vi "Protocol.Create Protocol Settings.vi"(8 "error in (no error)":errorcluster, 10 "Name in":string, 11 "Parameters in":T4={"Name"="", "XNET.Settings"={"Database"="", "Cluster"="", "Port"="", "Baud rate [Bd]"=0, "Termination"=0, "Incoming Decimation"=0, "Outgoing Decimation"=1}, "Monitor.Network"={"Address"=0, "Name"=0, "Include DA"=FALSE}, "Data"=[], "DTCs"=[], "Sim.Nodes.LUT"=variant, "Data.LUT"=variant, "PCL"=0} {"Monitor.Network"."Name" format="%.0x"; "DTCs"."Data"."DM1.Ref"."Data Reference" format="%.0x"; "DTCs"."Data"."DM1.Enable.Ref"."Data Reference" format="%.0x"; "DTCs"."Data"."DM2.Ref"."Data Reference" format="%.0x"; "DTCs"."Data"."DM2.Enable.Ref"."Data Reference" format="%.0x"; "Data"."Trigger.Refs"."Data Reference" format="%.0x"; "Data"."Disable.Refs"."Data Reference" format="%.0x"; "Data"."Timing.Refs"."Data Reference" format="%.0x"; "Data"."Network"."Name" format="%.0x"; "Data"."Incoming.Refs"."Data Reference" format="%.0x"; "Data"."Outgoing.Refs"."Data Reference" format="%.0x"; "XNET.Settings"."Termination" items=["Off", "On"]}) -> (0 "error out":errorcluster, 3 "Protocol Refs":T1)   [LabVIEW 2019, in "J1939 Addon Engine.lvlib"]
uses:
  J1939 Addon Engine.lvlib
  Types/Protocol.App Settings.ctl
  Addon Shared/Types/XNET Settings.ctl
  Addon Shared/Types/Monitor Settings.ctl
  Types/Protocol.XNET Refs.ctl
  <vilib>/NI VeriStand/Custom Device API/Block Data Reference.ctl
  <vilib>/NI VeriStand/Custom Device API/Data Reference.ctl
  Types/Main.Outgoing.Frame.Settings.ctl
  Addon Shared/Types/Outgoing Event Trigger Types.ctl
  SubModules/Frame Protection Support/Source/Shared/Types/Exported Frame Settings.ctl
  SubModules/Frame Protection Support/Source/Shared/Types/Exported Frame Type.ctl
  SubModules/Frame Protection Support/Source/Shared/Types/Exported Protection Settings.ctl
  SubModules/Frame Protection Support/Source/Shared/Types/Protection Type.ctl
  SubModules/Frame Protection Support/Source/Shared/Types/XNET Signal Configuration.ctl
  SubModules/Frame Protection Support/Source/Shared/Types/Exported Counter Settings.ctl
  SubModules/Frame Protection Support/Source/Shared/Types/Exported Event Trigger Type.ctl
  Types/Engine.DTC Settings.ctl
  Addon Shared/Types/Compiled Simulated Settings.ctl
  Types/Engine.DTC FIFOs.ctl
  Types/Protocol.Refs.ctl
  Support Libraries/J1939 Utilities/Types/CAN Outgoing Message Cluster.ctl
  Types/Protocol.RQST Lookup Table Reference.ctl
  Types/Protocol.Address Table Reference.ctl
  Support Libraries/J1939 Utilities/J1939 Utilities.lvlib
  Addon Shared/J1939 Addon Shared.lvlib
  <vilib>/NI VeriStand/Custom Device API/Custom Device API.lvlib
  SubModules/Frame Protection Support/Source/Shared/Protection and Counter Support Shared.lvlib
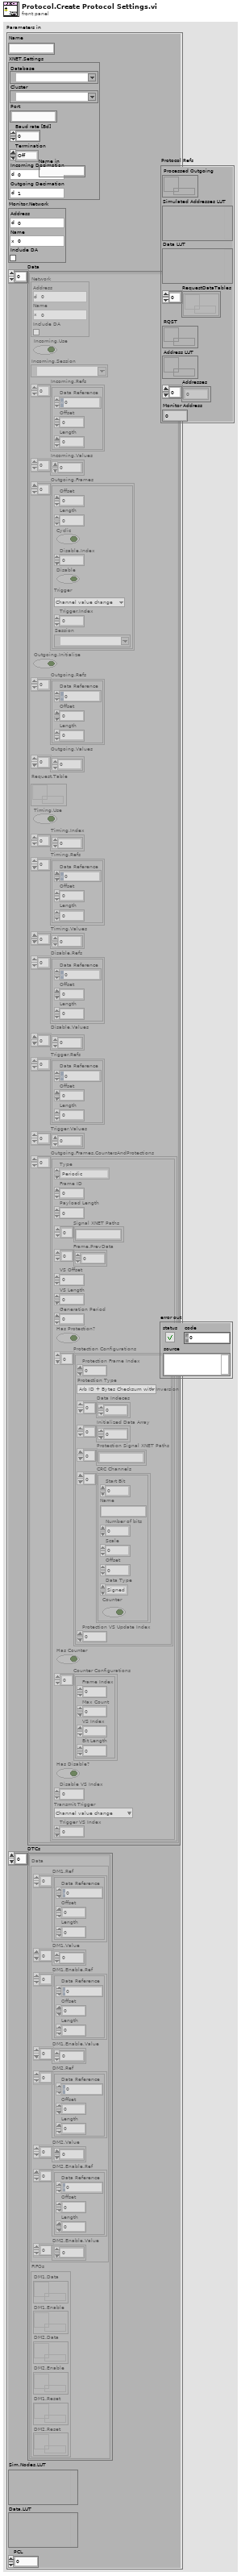
[diagram p1: front panel]
types:
  T1 = typedef "J1939 Addon Engine.lvlib/Protocol.Refs.ctl" = cluster{"Processed Outgoing":refnum<queue>, "Simulated Addresses LUT":variant, "Data LUT":variant, "RequestDataTables":refnum<k33>[], "RQST":T2, "Address LUT":T3, "Addresses":u8[], "Monitor Address":u8}
  T2 = typedef "J1939 Addon Engine.lvlib/Protocol.RQST Lookup Table Reference.ctl" = refnum<data-value>
  T3 = typedef "J1939 Addon Engine.lvlib/Protocol.Address Table Reference.ctl" = refnum<data-value>
  T4 = typedef "J1939 Addon Engine.lvlib/Protocol.App Settings.ctl" = cluster{"Name":string, "XNET.Settings":T5, "Monitor.Network":T6, "Data":T7[], "DTCs":T19[], "Sim.Nodes.LUT":variant, "Data.LUT":variant, "PCL":u32}
  T5 = typedef "J1939 Addon Shared.lvlib/XNET Settings.ctl" = cluster{"Database":refnum<k21>, "Cluster":refnum<k21>, "Port":string, "Baud rate [Bd]":u32, "Termination":u32, "Incoming Decimation":u32, "Outgoing Decimation":u32}
  T6 = typedef "J1939 Addon Shared.lvlib/Monitor Settings.ctl" = cluster{"Address":u8, "Name":u64, "Include DA":bool}
  T7 = typedef "J1939 Addon Engine.lvlib/Protocol.XNET Refs.ctl" = cluster{"Network":T6, "Incoming.Use":bool, "Incoming.Session":refnum<k21>, "Incoming.Refs":T8[], "Incoming.Values":dbl[], "Outgoing.Frames":T10[], "Outgoing.Initialize":bool, "Outgoing.Refs":T8[], "Outgoing.Values":dbl[], "Request.Table":refnum<k33>, "Timing.Use":bool, "Timing.Index":i32[], "Timing.Refs":T8[], "Timing.Values":dbl[], "Disable.Refs":T8[], "Disable.Values":dbl[], "Trigger.Refs":T8[], "Trigger.Values":dbl[], "Outgoing.Frames.CountersAndProtections":T12[]}
  T8 = typedef "Custom Device API.lvlib/Block Data Reference.ctl" = cluster{"Data Reference":T9, "Offset":u64, "Length":u64}
  T9 = typedef "Custom Device API.lvlib/Data Reference.ctl" = i32
  T10 = typedef "J1939 Addon Engine.lvlib/Main.Outgoing.Frame.Settings.ctl" = cluster{"Offset":u32, "Length":u32, "Cyclic":bool, "Disable.Index":i32, "Disable":bool, "Trigger":T11, "Trigger.Index":i32, "Session":refnum<k21>}
  T11 = typedef "J1939 Addon Shared.lvlib/Outgoing Event Trigger Types.ctl" = enum16{"Channel value change", "Trigger channel (not zero)", "Channel value change or trigger channel (not zero)", "Trigger channel (any value change)", "Channel value change or trigger channel (any value change)"}
  T12 = typedef "Protection and Counter Support Shared.lvlib/Exported Frame Settings.ctl" = cluster{"Type":T13, "Frame ID":u32, "Payload Length":u32, "Signal XNET Paths":string[], "Frame.PrevData":dbl[], "VS Offset":i32, "VS Length":i32, "Generation Period":u32, "Has Protection?":bool, "Protection Configurations":T14[], "Has Counter":bool, "Counter Configurations":T17[], "Has Disable?":bool, "Disable VS Index":i32, "Transmit Trigger":T18, "Trigger VS Index":i32}
  T13 = typedef "Protection and Counter Support Shared.lvlib/Exported Frame Type.ctl" = enum16{"Periodic", "Event", "Periodic/Event"}
  T14 = typedef "Protection and Counter Support Shared.lvlib/Exported Protection Settings.ctl" = cluster{"Protection Frame Index":i32, "Protection Type":T15, "Data Indeces":i32[], "Initialized Data Array":dbl[], "Protection Signal XNET Paths":string[], "CRC Channels":T16[], "Protection VS Update Index":i32}
  T15 = typedef "Protection and Counter Support Shared.lvlib/Protection Type.ctl" = enum16{"Arb ID + Bytes Checksum with Inversion", "Arb ID + Bytes CRC with Inversion", "Reversed Raw Signal Checksum with Inversion", "Concatenated Two's Compliment"}
  T16 = typedef "Protection and Counter Support Shared.lvlib/XNET Signal Configuration.ctl" = cluster{"Start Bit":i32, "Name":string, "Number of bits":i32, "Scale":dbl, "Offset":dbl, "Data Type":u32, "Counter":bool}
  T17 = typedef "Protection and Counter Support Shared.lvlib/Exported Counter Settings.ctl" = cluster{"Frame Index":i32, "Max Count":dbl, "VS Index":i32, "Bit Length":i64}
  T18 = typedef "Protection and Counter Support Shared.lvlib/Exported Event Trigger Type.ctl" = enum16{"Channel value change", "Trigger channel (not zero)", "Channel value change or trigger channel (not zero)", "Trigger channel (any value change)", "Channel value change or trigger channel (any value change)"}
  T19 = typedef "J1939 Addon Engine.lvlib/Engine.DTC Settings.ctl" = cluster{"Data":T20, "FIFOs":T21}
  T20 = typedef "J1939 Addon Shared.lvlib/Compiled Simulated Settings.ctl" = cluster{"DM1.Ref":T8[], "DM1.Value":dbl[], "DM1.Enable.Ref":T8[], "DM1.Enable.Value":dbl[], "DM2.Ref":T8[], "DM2.Value":dbl[], "DM2.Enable.Ref":T8[], "DM2.Enable.Value":dbl[]}
  T21 = typedef "J1939 Addon Engine.lvlib/Engine.DTC FIFOs.ctl" = cluster{"DM1.Data":refnum<k33>, "DM1.Enable":refnum<k33>, "DM2.Data":refnum<k33>, "DM2.Enable":refnum<k33>, "DM1.Reset":refnum<k33>, "DM2.Reset":refnum<k33>}
  T22 = typedef "J1939 Utilities.lvlib/CAN Outgoing Message Cluster.ctl" = cluster{"Identifier":u32, "Data":u8[]}
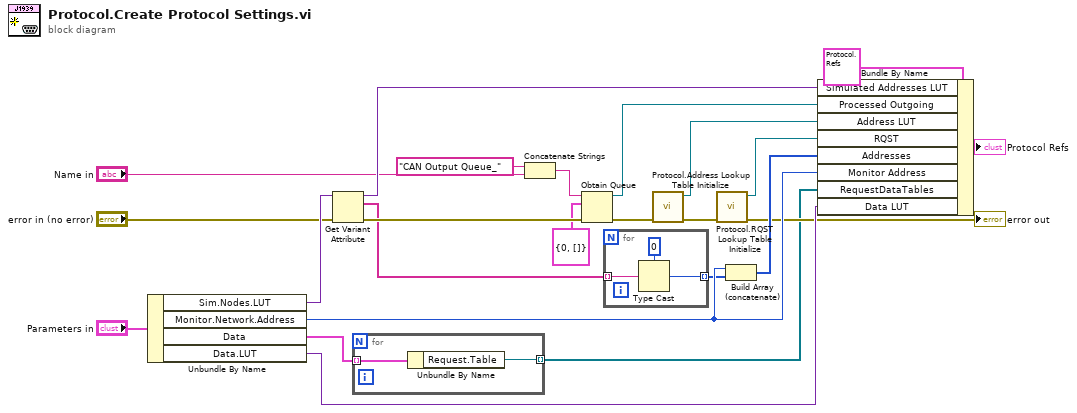
[diagram p0: block diagram]
diagram:
  n1 = Unbundle By Name("Parameters in") -> ("Sim.Nodes.LUT"=w20:variant, "Monitor.Network.Address"=w24:u8, "Data"=w22:T7[], "Data.LUT"=w21:variant)
  n2 = Get Variant Attribute(Variant=w20, error in="error in (no error)") -> (duplicate Variant=w23:variant, names=w2:string[], error out=w19:errorcluster)  [unwired: 2 in, 1 out]
  n3 = for {
    tunnel: w22 -> [w26] mode=indexing
    tunnel: [w25] -> w1 mode=indexing
    n4 = Unbundle By Name(w26) -> ("Request.Table"=w25:refnum<k33>)
  }
  n5 = Concatenate Strings("CAN Output Queue_" ("name (unnamed)"), "Name in") -> (w10:string)
  n6 = Obtain Queue(name (unnamed)=w10, element data type=T22 {"Identifier"=0, "Data"=[]} ("Data to Send"), error in (no error)=w19) -> (queue out=w12:refnum<queue>, error out=w4:errorcluster)  [unwired: 2 in, 1 out]
  n7 = for {
    tunnel: w2 -> [w29] mode=indexing
    tunnel: [w27] -> w3 mode=indexing
    n8 = Type Cast(type=u8 0, x=w29) -> (*(type *) &x=w27:u8)
  }
  n9 = call "Protocol.Address Lookup Table Initialize.vi"("error in (no error)"=w4) -> ("error out"=w5:errorcluster, "Address LUT"=w13:T3)  [unwired: 9 in]
  n10 = call "Protocol.RQST Lookup Table Initialize.vi"("error in (no error)"=w5) -> ("error out"=→"error out":errorcluster, "Rqst LUT"=w14:T2)  [unwired: 9 in]
  n11 = Build Array (concatenate)(w24, w3) -> (w15:u8[])
  n12 = Bundle By Name(cluster=T1 {"Processed Outgoing"=refnum, "Simulated Addresses LUT"=variant, "Data LUT"=variant, "RequestDataTables"=[], "RQST"=refnum, "Address LUT"=refnum, "Addresses"=[], "Monitor Address"=0} ("Protocol Refs"), "Simulated Addresses LUT"=w23, "Processed Outgoing"=w12, "Address LUT"=w13, "RQST"=w14, "Addresses"=w15, "Monitor Address"=w24, "RequestDataTables"=w1, "Data LUT"=w21) -> (→"Protocol Refs":T1)
